vi "Main-side_features.vi"() -> ()   [LabVIEW 2015]
uses:
  <vilib>/Analysis/baseanly.llb/Mean (DBL).vi
  <vilib>/Utility/file.llb/Read Delimited Spreadsheet (string).vi
  <vilib>/Utility/file.llb/Write Delimited Spreadsheet (string).vi
  <vilib>/vision/NI_Vision_Development_Module.lvlib
  PlantType.dll
  TotalContoursConvexHull.dll
  2-top_features_oilseed/HistProperty.dll
  <vilib>/Analysis/NI_AALBase.lvlib
panel:
  in  "title-Path":path=path "H:/3-side_features_oilseed/title.txt"
  out "Gray Image":T1(plugin-control)
  out "savePath":path
  out "appended array":string[](array[string])
  out "im_width":i32
  out "im_height":i32
  in  "Date Path":path=path "H:/3-side_features_oilseed/rape_test/path.txt"
  out "Current Path":path
  out "Current Number":string
  out "Rotated Image":T1(plugin-control)
  out "HistStat_whole":dbl[](array[numeric])
  out "PAR (perimeter-to-area ratio)":dbl
  out "SFD":sgl
  out "BW (minimum circumscribed box width)":dbl
  out "BH (minimum circumscribed box height)":dbl
  out "TPA (Total projective area)":dbl
  out "R (Rectangularity)":dbl
  out "IFD":sgl
  out "Hull area":dbl
  out "AC (Area Convexity)":dbl
  out "HWR":dbl
  in  "ROI_flower":T2={"Top"=0, "im_height"=1450, "L_left"=0, "im_width"=1680}
  out "NB (Number of blanchs)":i32
  out "FPAR (Flower perimeter-to-area ratio)":dbl
  out "FSFD":sgl
  out "FBW (Flower minimum circumscribed box width)":dbl
  out "FBH (Flower minimum circumscribed box height)":dbl
  out "YPA (Yellow projective area)":dbl
  out "FR (Flower rectangularity)":dbl
  out "FIFD":sgl
  out "FAC (Flower area Convexity)":dbl
  out "HistStat_flower":dbl[](array[numeric])
  in  "ROI_whole":T2={"Top"=90, "im_height"=1970, "L_left"=300, "im_width"=1450}
  out "FHWR":dbl
  out "GPA (Green projective area)":dbl
  out "GPAR (Green / Total)":dbl
  out "YPAR (Yellow / Total)":dbl
  out "Flower Hull Image":T1(plugin-control)
  out "Flower Hull Area":dbl
  out "Cropped Image":T1(plugin-control)
  out "Binary Image":T1(plugin-control)
  out "rgb Hull Image":T1(plugin-control)
  out "Flower Image (RGB)":T1(plugin-control)
  out "Flower Image (Label)":T1(plugin-control)
  out "PD1-6":sgl[](array[numeric])
  out "f array":dbl[](array[numeric])
  out "Combined Image":T1(plugin-control)
  out "Image Path":path
  in  "Image Main Path":path=path "H:/3-side_features_oilseed/rape_test"
  # "Digital evaluation software for oilseed rape \nphenotype-related traits (side-view)"
  # "测量数据"
  # "Whole plant"
  # "均值"
  # "标准差"
  # "平滑度"
  # "三阶矩"
  # "一致性"
  # "熵"
  # "Flower"
  # "Ratio"
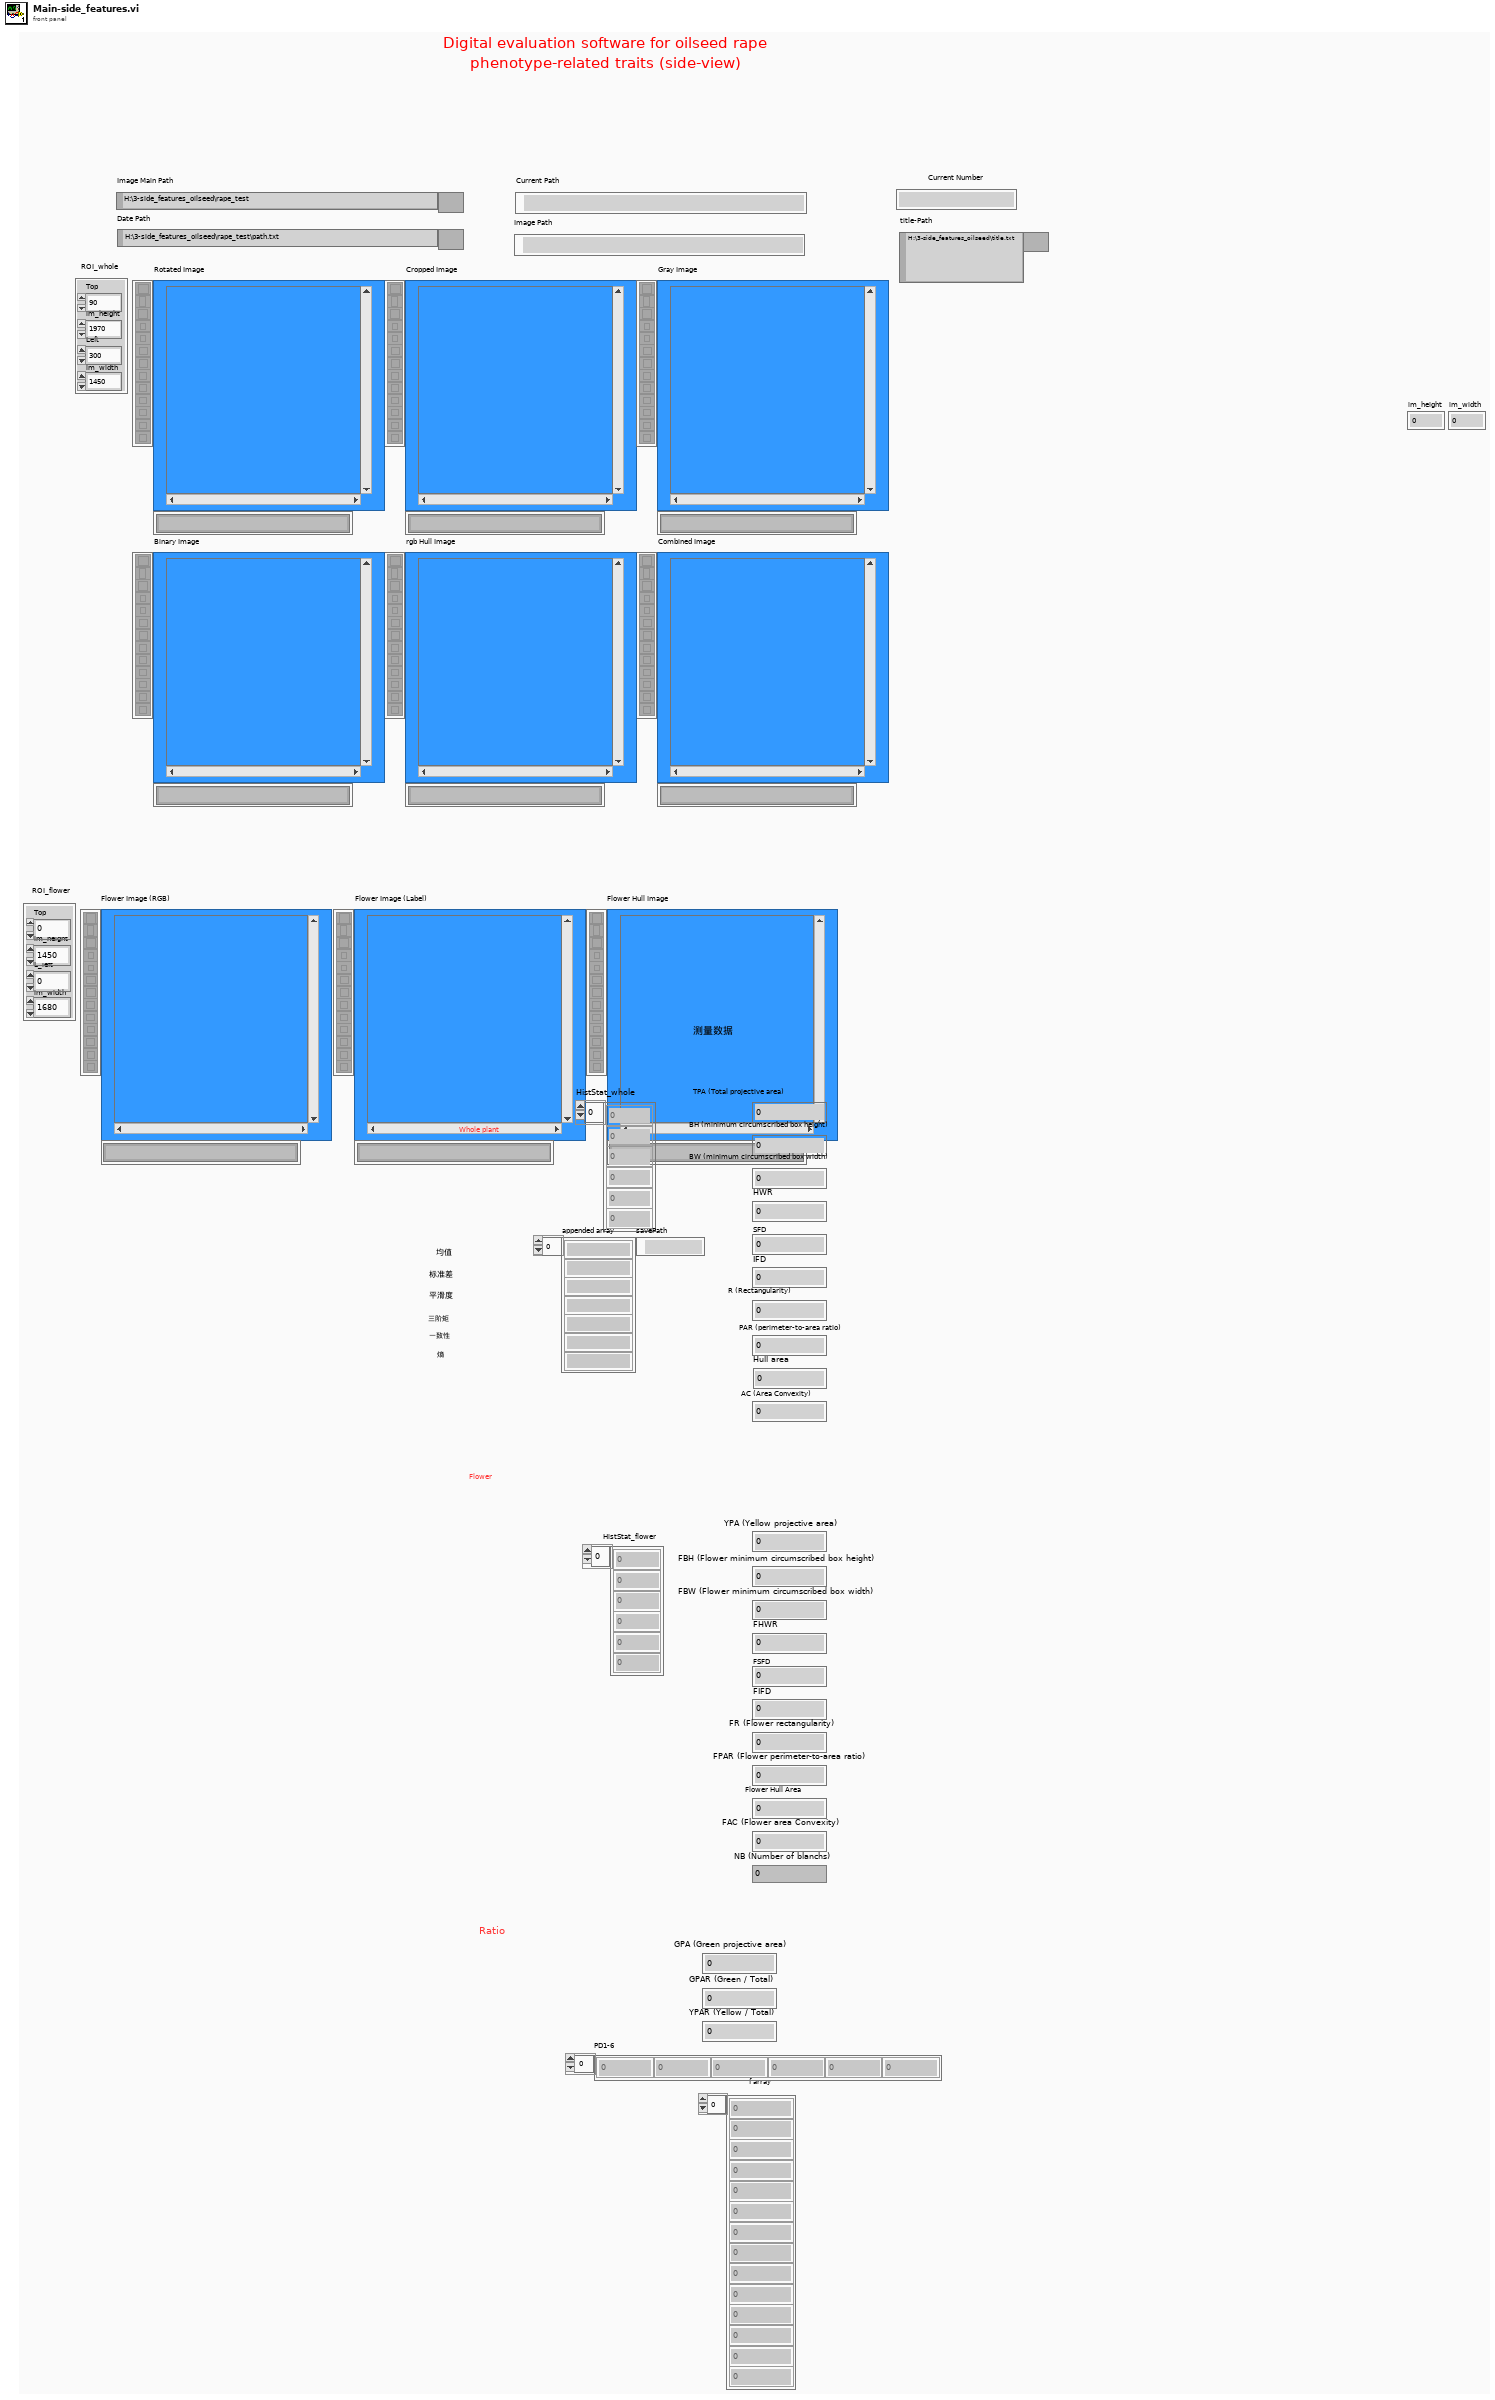
[diagram p1: front panel]
types:
  T1 = typedef "IMAQ Image.ctl" = refnum<image>
  T2 = cluster{"Top":i32, "im_height":i32, "L_left":i32, "im_width":i32}
  T3 = typedef "Image Type" = u32
  T4 = typedef "Particle Parameters" = i32
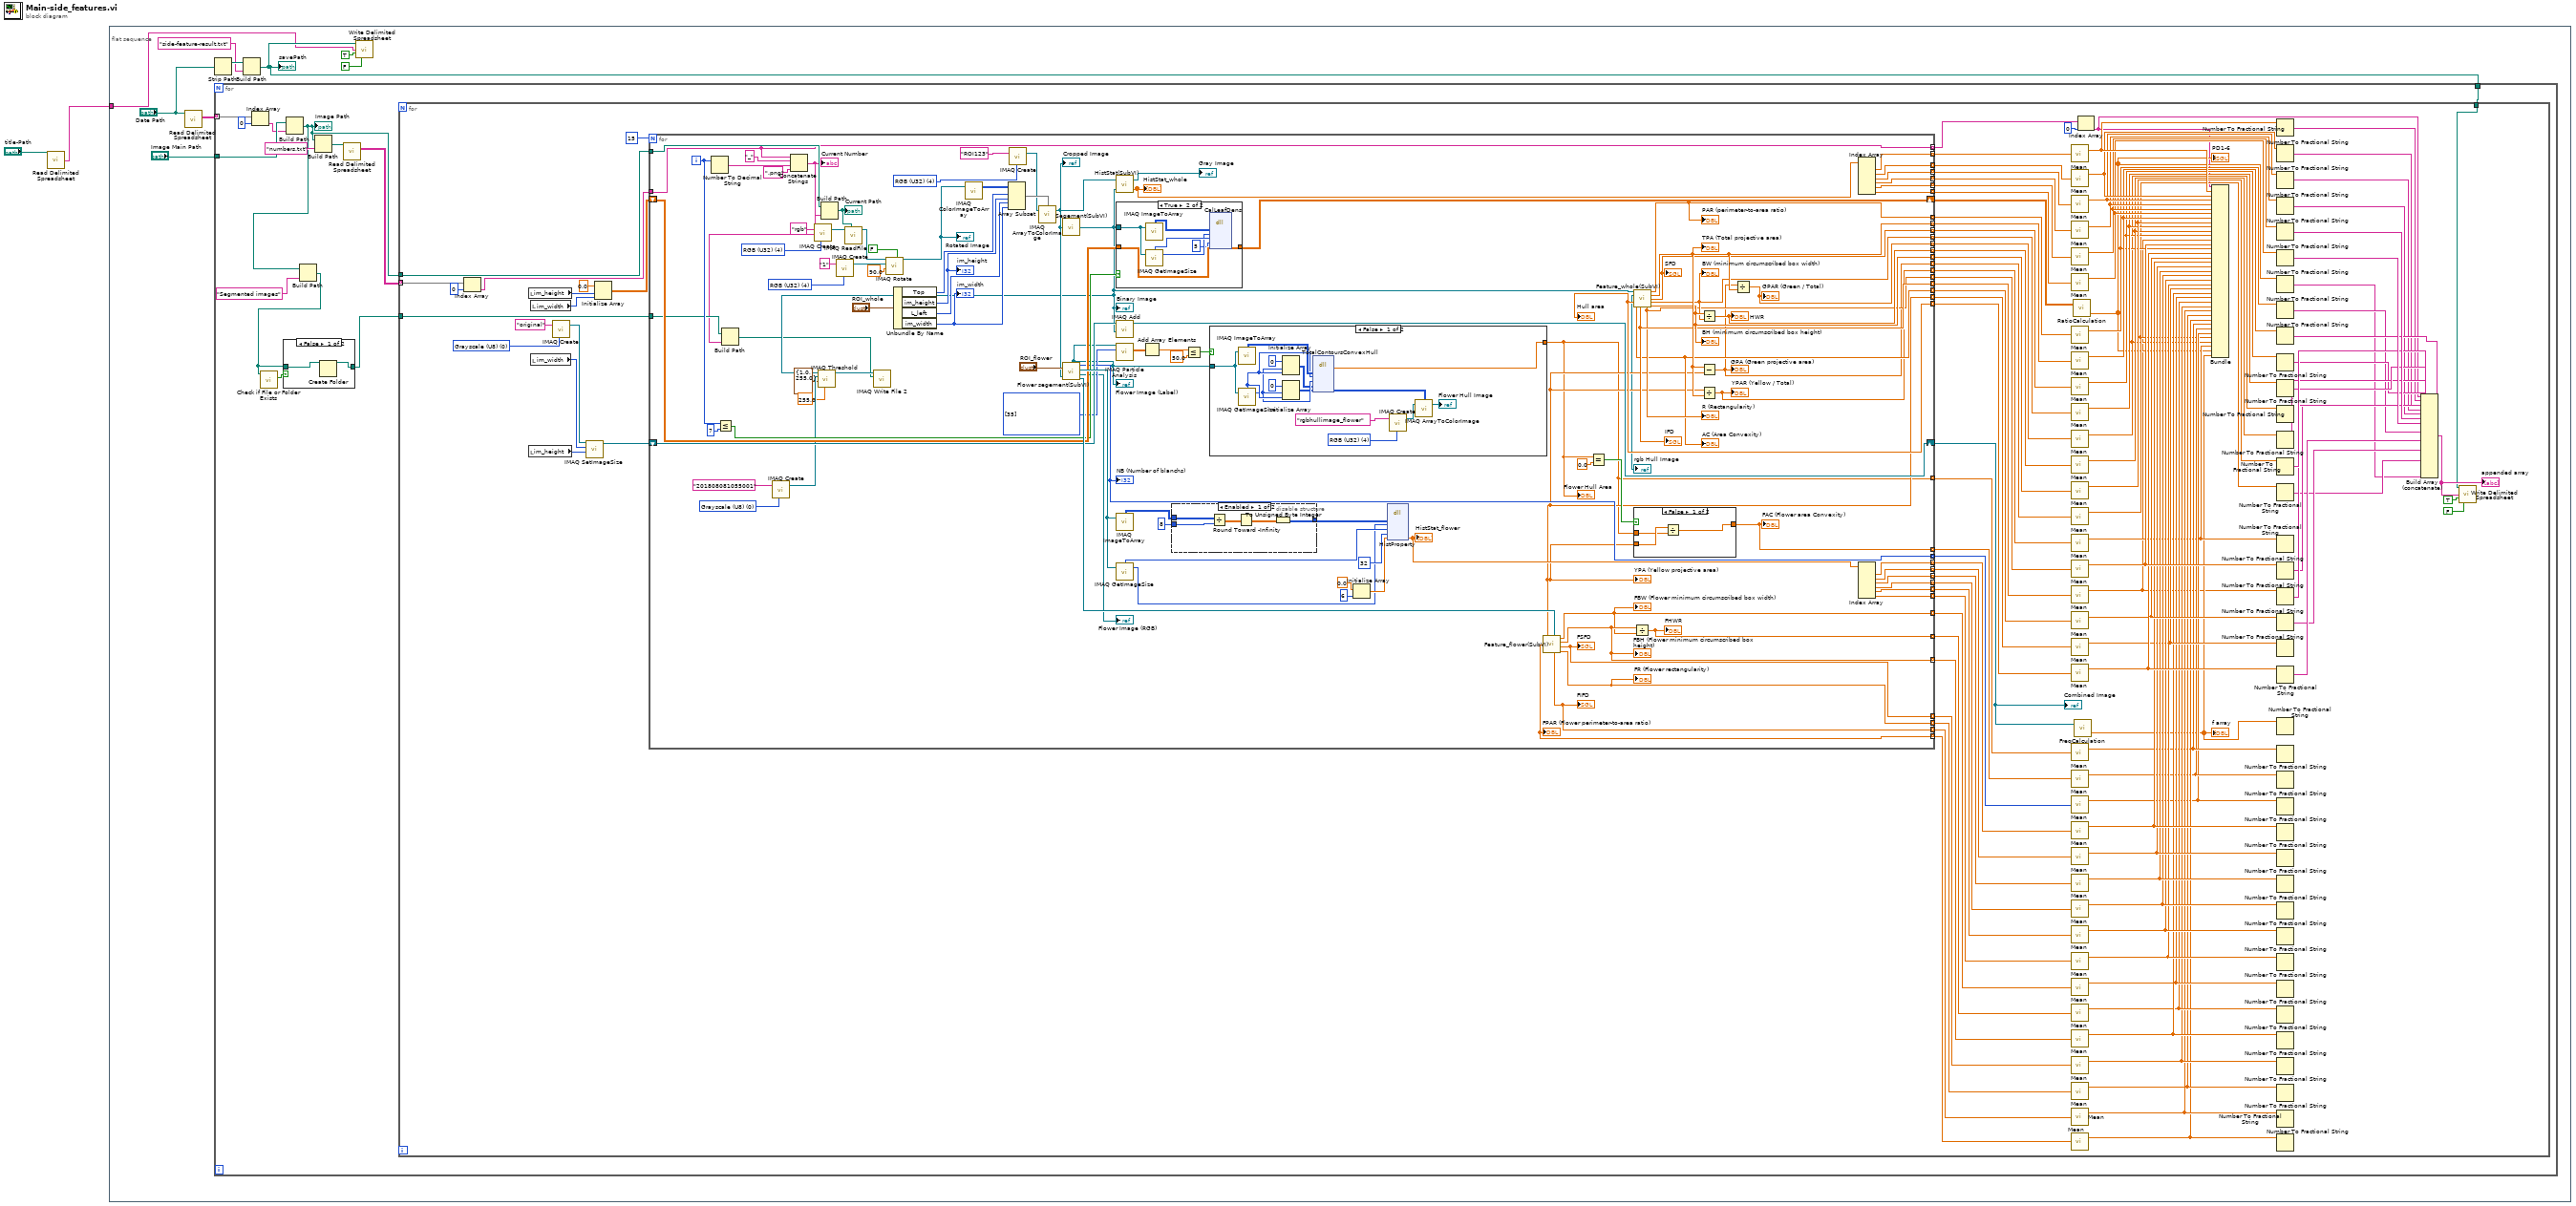
[diagram p0: block diagram]
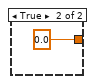
[diagram p3: hidden frame]
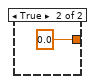
[diagram p4: hidden frame]
diagram:
  n1 = call-poly <vilib>:"Read Delimited Spreadsheet.vi"("file path (dialog if empty)"="title-Path") -> ("first row"=w1:string[])  [unwired: 9 in, 5 out]
  n2 = flat-sequence {
    tunnel: w1 -> [w3]
    frame #0 {
      n3 = call-poly <vilib>:"Read Delimited Spreadsheet.vi"("file path (dialog if empty)"="Date Path") -> ("all rows"=w10:string[][])  [unwired: 9 in, 5 out]
      n4 = Strip Path(path="Date Path") -> (stripped path=w8:path)  [unwired: 1 out]
      n5 = Build Path(base path=w8, name or relative path="side-feature-result.txt") -> (appended path=w4:path)
      "savePath" <- w4
      n6 = for {
        tunnel: "Image Main Path" -> [w24]
        tunnel: w10 -> [w22] mode=indexing
        tunnel: w4 -> [w17]
        n7 = Index Array(array=w22, index=0) -> (element=w19:string)
        n8 = Build Path(base path=w24, name or relative path=w19) -> (appended path=w16:path)
        "Image Path" <- w16
        n9 = Build Path(base path=w16, name or relative path="Segmented images") -> (appended path=w13:path)
        n10 = call <vilib>:"Check if File or Folder Exists.vi"("path"=w13) -> ("file or folder exists?"=w14:bool)  [unwired: 8 in, 2 out]
        n11 = case shown="False" w14 {
          tunnel: [w25 w27] -> w12
          tunnel: w13 -> [w26 w27]
          frame False {
            n12 = Create Folder(path (use dialog)=w26) -> (created path=w25:path)  [unwired: 2 in, 2 out]
          }
          frame True {
          }
        }
        n13 = Build Path(base path=w16, name or relative path="numbers.txt") -> (appended path=w20:path)
        n14 = call-poly <vilib>:"Read Delimited Spreadsheet.vi"("file path (dialog if empty)"=w20) -> ("all rows"=w18:string[][])  [unwired: 9 in, 5 out]
        n15 = for {
          tunnel: w16 -> [w142]
          tunnel: w18 -> [w143] mode=indexing
          tunnel: w17 -> [w32]
          tunnel: w12 -> [w31]
          w134 = T3 0 items=["Grayscale (U8)", "Grayscale (I16)", "Grayscale (SGL)", "Complex (CSG)", "RGB (U32)", "HSL (U32)", "RGB (U64)", "Grayscale (U16)"] ("Image Type")
          n16 = Index Array(array=w143, index=0) -> (element=w141:string)
          n17 = local read "im_height"() -> (w93:i32)
          n18 = local read "im_height"() -> (w92:i32)
          n19 = local read "im_width"() -> (w91:i32)
          n20 = local read "im_width"() -> (w90:i32)
          n21 = call "IMAQ Create"("Image Name"="original", "Image Type"=w134) -> ("New Image"=w135:T1)  [unwired: 2 in, 2 out]
          n22 = call "IMAQ SetImageSize"("Y Resolution"=w92, "X Resolution"=w90, "Image"=w135) -> ("Image Out"=w133:T1)  [unwired: 1 in, 2 out]
          n23 = Initialize Array(sgl 0.0 ("element"), w93, w91) -> (w138:sgl[][])
          n24 = for {
            N: 15 -> [_]
            tunnel: w142 -> [w242]
            tunnel: w141 -> [w157]
            shift-right: [w209] -> w137
            shift-left: w138 -> [w212]
            shift-right: [w207] -> w96
            shift-left: w133 -> [w208]
            tunnel: [w205] -> w132 mode=indexing
            tunnel: [w204] -> w131 mode=indexing
            tunnel: [w203] -> w130 mode=indexing
            tunnel: [w202] -> w129 mode=indexing
            tunnel: [w201] -> w128 mode=indexing
            tunnel: [w200] -> w127 mode=indexing
            tunnel: [w199] -> w126 mode=indexing
            tunnel: [w198] -> w125 mode=indexing
            tunnel: [w197] -> w124 mode=indexing
            tunnel: [w196] -> w123 mode=indexing
            tunnel: [w195] -> w122 mode=indexing
            tunnel: [w194] -> w121 mode=indexing
            tunnel: [w193] -> w120 mode=indexing
            tunnel: [w192] -> w119 mode=indexing
            tunnel: [w191] -> w118 mode=indexing
            tunnel: [w190] -> w117 mode=indexing
            tunnel: [w188] -> w116 mode=indexing
            tunnel: [w187] -> w115 mode=indexing
            tunnel: [w186] -> w114 mode=indexing
            tunnel: [w185] -> w113 mode=indexing
            tunnel: [w184] -> w112 mode=indexing
            tunnel: [w183] -> w111 mode=indexing
            tunnel: [w164] -> w110 mode=indexing
            tunnel: [w182] -> w109 mode=indexing
            tunnel: [w181] -> w108 mode=indexing
            tunnel: [w180] -> w107 mode=indexing
            tunnel: [w179] -> w106 mode=indexing
            tunnel: [w178] -> w105 mode=indexing
            tunnel: [w177] -> w104 mode=indexing
            tunnel: [w176] -> w103 mode=indexing
            tunnel: [w163] -> w102 mode=indexing
            tunnel: [w162] -> w101 mode=indexing
            tunnel: [w175] -> w100 mode=indexing
            tunnel: [w174] -> w99 mode=indexing
            tunnel: [w173] -> w98 mode=indexing
            tunnel: [w172] -> w97 mode=indexing
            tunnel: [w157] -> w95 mode=indexing
            tunnel: w31 -> [w154]
            i -> [w156]
            w150 = u32 0 items=["Grayscale (U8)", "Grayscale (I16)", "Grayscale (SGL)", "Complex (CSG)", "RGB (U32)", "HSL (U32)", "RGB (U64)"] ("Image Type")
            w171 = T4[] [35] items=["Center of Mass X", "Center of Mass Y", "First Pixel X", "First Pixel Y", "Bounding Rect Left", "Bounding Rect Top", "Bounding Rect Right", "Bounding Rect Bottom", "Max Feret Diameter Start X", "Max Feret Diameter Start Y", "Max Feret Diameter End X", "Max Feret Diameter End Y", "Max Horiz. Segment Length Left", "Max Horiz. Segment Length Right", "Max Horiz. Segment Length Row", "-", "Bounding Rect Width", "Bounding Rect Height", "Bounding Rect Diagonal", "Perimeter", "Convex Hull Perimeter", "Holes' Perimeter", "Max Feret Diameter", "Equivalent Ellipse Major Axis", "Equivalent Ellipse Minor Axis", "Equivalent Ellipse Minor Axis (Feret)", "Equivalent Rect Long Side", "Equivalent Rect Short Side", "Equivalent Rect Diagonal", "Equivalent Rect Short Side (Feret)", "Average Horiz. Segment Length", "Average Vert. Segment Length", "Hydraulic Radius", "Waddel Disk Diameter", "-", "Area", "Holes' Area", "Particle & Holes' Area", "Convex Hull Area", "Image Area", "-", "Number of Holes", "Number of Horiz. Segments", "Number of Vert. Segments", "-", "Orientation", "Max Feret Diameter Orientation", "-", "% Area/Image Area", "% Area/(Particle & Holes' Area)", "Ratio of Equivalent Ellipse Axes", "Ratio of Equivalent Rect Sides", "-", "Elongation Factor", "Compactness Factor", "Heywood Circularity Factor", "Type Factor", "-", "Sum X", "Sum Y", "Sum XX", "Sum XY", "Sum YY", "Sum XXX", "Sum XXY", "Sum XYY", "Sum YYY", "-", "Moment of Inertia XX", "Moment of Inertia XY", "Moment of Inertia YY", "Moment of Inertia XXX", "Moment of Inertia XXY", "Moment of Inertia XYY", "Moment of Inertia YYY", "Norm. Moment of Inertia XX", "Norm. Moment of Inertia XY", "Norm. Moment of Inertia YY", "Norm. Moment of Inertia XXX", "Norm. Moment of Inertia XXY", "Norm. Moment of Inertia XYY", "Norm. Moment of Inertia YYY", "Hu Moment 1", "Hu Moment 2", "Hu Moment 3", "Hu Moment 4", "Hu Moment 5", "Hu Moment 6", "Hu Moment 7"] ("Pixel Measurements")
            w228 = u32 4 items=["Grayscale (U8)", "Grayscale (I16)", "Grayscale (SGL)", "Complex (CSG)", "RGB (U32)", "HSL (U32)", "RGB (U64)"] ("Image Type")
            w240 = T3 4 items=["Grayscale (U8)", "Grayscale (I16)", "Grayscale (SGL)", "Complex (CSG)", "RGB (U32)", "HSL (U32)", "RGB (U64)", "Grayscale (U16)"] ("Image Type")
            w247 = T3 4 items=["Grayscale (U8)", "Grayscale (I16)", "Grayscale (SGL)", "Complex (CSG)", "RGB (U32)", "HSL (U32)", "RGB (U64)", "Grayscale (U16)"] ("Image Type")
            n25 = Number To Decimal String(number=w156) -> (decimal integer string=w244:string)  [unwired: 1 out]
            n26 = Less Or Equal?(x=w156, y=u32 7) -> (x <= y?=w210:bool)
            n27 = call "IMAQ Create"("Image Name"="201808081055001", "Image Type"=w150) -> ("New Image"=w149:T1)  [unwired: 2 in, 2 out]
            n28 = Concatenate Strings(w157, "_" ("string"), w244, ".png" ("string")) -> (w153:string)
            "Current Number" <- w153
            n29 = Build Path(base path=w154, name or relative path=w153) -> (appended path=w145:path)
            n30 = call "IMAQ Create"("Image Name"="rgb", "Image Type"=w247) -> ("New Image"=w248:T1)  [unwired: 2 in, 2 out]
            n31 = Build Path(base path=w242, name or relative path=w153) -> (appended path=w243:path)
            "Current Path" <- w243
            n32 = call "IMAQ Create"("Image Name"="1", "Image Type"=w240) -> ("New Image"=w238:T1)  [unwired: 2 in, 2 out]
            n33 = call "IMAQ ReadFile"("File Path"=w243, "Image"=w248) -> ("Image Out"=w236:T1)  [unwired: 3 in, 6 out]
            n34 = call "IMAQ Rotate"("Maintain Size"=FALSE, "Angle (degrees)"=sgl 90.0, "Image Dst"=w238, "Image Src"=w236) -> ("Image Dst Out"=w226:T1)  [unwired: 4 in, 3 out]
            "Rotated Image" <- w226
            n35 = Unbundle By Name("ROI_whole") -> ("Top"=w232:i32, "im_height"=w233:i32, "L_left"=w234:i32, "im_width"=w235:i32)
            "im_height" <- w233
            "im_width" <- w235
            n36 = call "IMAQ ColorImageToArray"("Image"=w226) -> ("Image Pixels (U32)"=w231:u32[][])  [unwired: 2 in, 3 out]
            n37 = Array Subset(array=w231, index (row)=w232, length (row)=w233, index (col)=w234, length (col)=w235) -> (w230:u32[][])
            n38 = call "IMAQ Create"("Image Name"="ROI123", "Image Type"=w228) -> ("New Image"=w227:T1)  [unwired: 2 in, 2 out]
            n39 = call "IMAQ ArrayToColorImage"("Image Pixels (U32)"=w230, "Image"=w227) -> ("Image Out"=w161:T1)  [unwired: 2 in, 2 out]
            "Cropped Image" <- w161
            n40 = call "Segement(SubVI).vi"("Image in"=w161) -> ("Binary Image"=w152:T1)
            "Binary Image" <- w152
            n41 = call "IMAQ Threshold"("Replace Value"=sgl 255.0, "Range"=cluster{"Lower value":sgl, "Upper value":sgl} {"Lower value"=1.0, "Upper value"=255.0}, "Image Dst"=w149, "Image Src"=w152) -> ("Image Dst Out"=w146:T1)  [unwired: 6 in, 1 out]
            n42 = call-poly "IMAQ Write File 2"("File Path"=w145, "Image"=w146) -> ()  [unwired: 8 in, 2 out]
            n43 = call "Flower segement(SubVI).vi"("Image in"=w161, "ROI 上半部分 2"="ROI_flower") -> ("黄色分量（油菜花）二值图"=w224:T1, "黄色分量（油菜花）"=→"Flower Image (RGB)":T1, "黄色分量（油菜花）Gray"=w214:T1, "Number of Particles"=w175:i32, "RGB花标记"=w158:T1)
            "NB (Number of blanchs)" <- w175
            "Flower Image (Label)" <- w158
            n44 = call "HistStat(SubVI).vi"("Binary Image"=w152, "Original Image"=w161) -> ("HistStat"=w206:dbl[], "Gray Image"=→"Gray Image":T1)
            "HistStat_whole" <- w206
            n45 = case shown="True" w210 {
              tunnel: w152 -> [_ w273]
              tunnel: w212 -> [w269 w272]
              tunnel: [w269 w271] -> w209
              frame False {
              }
              frame True {
                n46 = call "IMAQ ImageToArray"("Image"=w273) -> ("Image Pixels (U8)"=w276:u8[][])  [unwired: 2 in, 5 out]
                n47 = call "IMAQ GetImageSize"("Image"=w273) -> ("Y Resolution"=w274:i32, "X Resolution"=w275:i32)  [unwired: 1 in, 3 out]
                n48 = dll-call lib="H:/3-side_features_oilseed/PlantType.dll" fn="CalLeafDens"("bw"=w276, "row"=w274, "col"=w275, "GridSize"=5, "dens"=w272) -> ("dens"=w271:sgl[][])  [unwired: 7 in, 3 out]
              }
            }
            n49 = call "IMAQ Add"("Image Src A"=w208, "Image Src B"=w152) -> ("Image Dst Out"=w207:T1)  [unwired: 3 in, 3 out]
            n50 = call "IMAQ Particle Analysis"("Pixel Measurements"=w171, "Image"=w158) -> ("Particle Measurements (Pixels)"=w170:dbl[][])  [unwired: 3 in, 6 out]
            n51 = call "IMAQ ImageToArray"("Image"=w214) -> ("Image Pixels (U8)"=w215:u8[][])  [unwired: 2 in, 5 out]
            n52 = call "IMAQ GetImageSize"("Image"=w214) -> ("Y Resolution"=w218:i32, "X Resolution"=w219:i32)  [unwired: 1 in, 3 out]
            n53 = Add Array Elements(numeric array=w170) -> (sum=w169:dbl)
            n54 = disable-structure shown="Enabled" {
              disable-tunnel: w215 -> [w281 w282]
              disable-tunnel: u8 8 ("y") -> [w280 _]
              disable-tunnel: [w277 w282] -> w217
              frame Enabled {
                n55 = Divide(x=w281, y=w280) -> (x/y=w279:dbl[][])
                n56 = Round Toward -Infinity(1:w279) -> (0:w278:dbl[][])
                n57 = To Unsigned Byte Integer(number=w278) -> (unsigned 8bit integer=w277:u8[][])
              }
              frame Disabled {
              }
            }
            n58 = Less Or Equal?(x=w169, y=50.0) -> (x <= y?=w167:bool)
            n59 = case shown="False" w167 {
              tunnel: w158 -> [w256 _]
              tunnel: [w255 0.0 ("areaSum")] -> w163
              frame False {
                w262 = T3 4 items=["Grayscale (U8)", "Grayscale (I16)", "Grayscale (SGL)", "Complex (CSG)", "RGB (U32)", "HSL (U32)", "RGB (U64)", "Grayscale (U16)"] ("Image Type")
                n60 = call "IMAQ ImageToArray"("Image"=w256) -> ("Image Pixels (U8)"=w267:u8[][])  [unwired: 2 in, 5 out]
                n61 = call "IMAQ GetImageSize"("Image"=w256) -> ("Y Resolution"=w265:i32, "X Resolution"=w266:i32)  [unwired: 1 in, 3 out]
                n62 = Initialize Array(u8 0 ("element"), w265, w266) -> (w257:u8[][])
                n63 = Initialize Array(u32 0 ("element"), w265, w266) -> (w260:u32[][])
                n64 = dll-call lib="H:/3-side_features_oilseed/TotalContoursConvexHull.dll" fn="TotalContoursConvexHull"("src"=w267, "width"=w266, "height"=w265, "bwhullimage"=w257, "rgbhullimage"=w260) -> ("areaSum"=w255:dbl, "rgbhullimage"=w263:u32[][])  [unwired: 7 in, 2 out]
                n65 = call "IMAQ Create"("Image Name"="rgbhullimage_flower", "Image Type"=w262) -> ("New Image"=w264:T1)  [unwired: 2 in, 2 out]
                n66 = call "IMAQ ArrayToColorImage"("Image Pixels (U32)"=w263, "Image"=w264) -> ("Image Out"=→"Flower Hull Image":T1)  [unwired: 2 in, 2 out]
              }
              frame True {
              }
            }
            "Flower Hull Area" <- w163
            n67 = Initialize Array(0.0 ("element"), 6 ("dimension size")) -> (w222:dbl[])
            n68 = dll-call lib="H:/2-top_features_oilseed/HistProperty.dll" fn="HistProperty"("Im"=w217, "row"=w218, "col"=w219, "G"=32, "HistStat"=w222) -> ("HistStat"=w189:dbl[])  [unwired: 7 in, 3 out]
            "HistStat_flower" <- w189
            n69 = call "Feature_flower(SubVI).vi"("黄色分量（油菜花）二值图"=w224) -> ("SF 3"=w177:dbl, "IFD 2"=w178:sgl, "SFD 2"=w179:sgl, "SH 2"=w182:dbl, "SW 2"=w181:dbl, "SE 2"=w176:dbl, "SA"=w164:dbl)  [unwired: 1 out]
            "FPAR (Flower perimeter-to-area ratio)" <- w176
            "FSFD" <- w179
            "FBW (Flower minimum circumscribed box width)" <- w181
            "FBH (Flower minimum circumscribed box height)" <- w182
            "YPA (Yellow projective area)" <- w164
            "FR (Flower rectangularity)" <- w177
            "FIFD" <- w178
            n70 = Equal?(x=w163, y=0.0) -> (x = y?=w166:bool)
            n71 = Divide(x=w182, y=w181) -> (x/y=w180:dbl)
            "FHWR" <- w180
            n72 = call "Feature_whole(SubVI).vi"("Binary Image"=w152) -> ("SE"=w192:dbl, "rgb Hull Image 2"=→"rgb Hull Image":T1, "SA"=w199:dbl, "SFD"=w195:sgl, "Hull area"=w191:dbl, "SW"=w197:dbl, "SF 2"=w190:dbl, "IFD"=w194:sgl, "SF"=w193:dbl, "SH"=w198:dbl)  [unwired: 5 out]
            "PAR (perimeter-to-area ratio)" <- w192
            "SFD" <- w195
            "BW (minimum circumscribed box width)" <- w197
            "BH (minimum circumscribed box height)" <- w198
            "TPA (Total projective area)" <- w199
            "R (Rectangularity)" <- w193
            "IFD" <- w194
            "Hull area" <- w191
            "AC (Area Convexity)" <- w190
            n73 = case shown="False" w166 {
              tunnel: w164 -> [w252 _]
              tunnel: w163 -> [w251 _]
              tunnel: [w250 0.0] -> w162
              frame False {
                n74 = Divide(x=w252, y=w251) -> (x/y=w250:dbl)
              }
              frame True {
              }
            }
            "FAC (Flower area Convexity)" <- w162
            n75 = Divide(x=w198, y=w197) -> (x/y=w196:dbl)
            "HWR" <- w196
            n76 = Subtract(x=w199, y=w164) -> (x-y=w174:dbl)
            "GPA (Green projective area)" <- w174
            n77 = Divide(x=w164, y=w199) -> (x/y=w172:dbl)
            "YPAR (Yellow / Total)" <- w172
            n78 = Divide(x=w174, y=w199) -> (x/y=w173:dbl)
            "GPAR (Green / Total)" <- w173
            n79 = Index Array(array=w206) -> (element #1=w205:dbl, element #2=w204:dbl, element #3=w203:dbl, element #4=w202:dbl, element #5=w201:dbl, element #6=w200:dbl)  [unwired: 6 in]
            n80 = Index Array(array=w189) -> (element #1=w188:dbl, element #2=w187:dbl, element #3=w186:dbl, element #4=w185:dbl, element #5=w184:dbl, element #6=w183:dbl)  [unwired: 6 in]
          }
          "Combined Image" <- w96
          n81 = call-poly <vilib>:"Mean.vi"("X"=w132) -> ("mean"=w89:dbl)  [unwired: 1 out]
          n82 = call-poly <vilib>:"Mean.vi"("X"=w131) -> ("mean"=w88:dbl)  [unwired: 1 out]
          n83 = call-poly <vilib>:"Mean.vi"("X"=w130) -> ("mean"=w87:dbl)  [unwired: 1 out]
          n84 = call-poly <vilib>:"Mean.vi"("X"=w129) -> ("mean"=w86:dbl)  [unwired: 1 out]
          n85 = call-poly <vilib>:"Mean.vi"("X"=w128) -> ("mean"=w85:dbl)  [unwired: 1 out]
          n86 = call-poly <vilib>:"Mean.vi"("X"=w127) -> ("mean"=w84:dbl)  [unwired: 1 out]
          n87 = call-poly <vilib>:"Mean.vi"("X"=w119) -> ("mean"=w77:dbl)  [unwired: 1 out]
          n88 = call-poly <vilib>:"Mean.vi"("X"=w126) -> ("mean"=w83:dbl)  [unwired: 1 out]
          n89 = call-poly <vilib>:"Mean.vi"("X"=w122) -> ("mean"=w79:dbl)  [unwired: 1 out]
          n90 = call-poly <vilib>:"Mean.vi"("X"=w124) -> ("mean"=w81:dbl)  [unwired: 1 out]
          n91 = call-poly <vilib>:"Mean.vi"("X"=w98) -> ("mean"=w56:dbl)  [unwired: 1 out]
          n92 = call-poly <vilib>:"Mean.vi"("X"=w123) -> ("mean"=w80:dbl)  [unwired: 1 out]
          n93 = call-poly <vilib>:"Mean.vi"("X"=w125) -> ("mean"=w82:dbl)  [unwired: 1 out]
          n94 = call-poly <vilib>:"Mean.vi"("X"=w99) -> ("mean"=w57:dbl)  [unwired: 1 out]
          n95 = call-poly <vilib>:"Mean.vi"("X"=w97) -> ("mean"=w55:dbl)  [unwired: 1 out]
          n96 = call-poly <vilib>:"Mean.vi"("X"=w120) -> ("mean"=w78:dbl)  [unwired: 1 out]
          n97 = call-poly <vilib>:"Mean.vi"("X"=w121) -> ("mean"=w28:dbl)  [unwired: 1 out]
          n98 = call-poly <vilib>:"Mean.vi"("X"=w117) -> ("mean"=w75:dbl)  [unwired: 1 out]
          n99 = call-poly <vilib>:"Mean.vi"("X"=w110) -> ("mean"=w68:dbl)  [unwired: 1 out]
          n100 = call-poly <vilib>:"Mean.vi"("X"=w118) -> ("mean"=w76:dbl)  [unwired: 1 out]
          n101 = call-poly <vilib>:"Mean.vi"("X"=w102) -> ("mean"=w60:dbl)  [unwired: 1 out]
          n102 = call-poly <vilib>:"Mean.vi"("X"=w101) -> ("mean"=w59:dbl)  [unwired: 1 out]
          n103 = call-poly <vilib>:"Mean.vi"("X"=w100) -> ("mean"=w58:dbl)  [unwired: 1 out]
          n104 = call-poly <vilib>:"Mean.vi"("X"=w116) -> ("mean"=w74:dbl)  [unwired: 1 out]
          n105 = call-poly <vilib>:"Mean.vi"("X"=w115) -> ("mean"=w73:dbl)  [unwired: 1 out]
          n106 = call-poly <vilib>:"Mean.vi"("X"=w114) -> ("mean"=w72:dbl)  [unwired: 1 out]
          n107 = call-poly <vilib>:"Mean.vi"("X"=w113) -> ("mean"=w71:dbl)  [unwired: 1 out]
          n108 = call-poly <vilib>:"Mean.vi"("X"=w112) -> ("mean"=w70:dbl)  [unwired: 1 out]
          n109 = call-poly <vilib>:"Mean.vi"("X"=w111) -> ("mean"=w69:dbl)  [unwired: 1 out]
          n110 = call-poly <vilib>:"Mean.vi"("X"=w108) -> ("mean"=w66:dbl)  [unwired: 1 out]
          n111 = call-poly <vilib>:"Mean.vi"("X"=w107) -> ("mean"=w65:dbl)  [unwired: 1 out]
          n112 = call-poly <vilib>:"Mean.vi"("X"=w109) -> ("mean"=w67:dbl)  [unwired: 1 out]
          n113 = call-poly <vilib>:"Mean.vi"("X"=w106) -> ("mean"=w64:dbl)  [unwired: 1 out]
          n114 = call-poly <vilib>:"Mean.vi"("X"=w104) -> ("mean"=w62:dbl)  [unwired: 1 out]
          n115 = call-poly <vilib>:"Mean.vi"("X"=w105) -> ("mean"=w63:dbl)  [unwired: 1 out]
          n116 = call-poly <vilib>:"Mean.vi"("X"=w103) -> ("mean"=w61:dbl)  [unwired: 1 out]
          n117 = call "RatioCalculation.vi"("dens"=w137) -> ("ratio"=w54:sgl[])  [unwired: 2 out]
          "PD1-6" <- w54
          n118 = call "FreqCalculation.vi"("Acc Image"=w96) -> ("f array"=w53:dbl[])  [unwired: 2 out]
          "f array" <- w53
          n119 = Index Array(array=w95, index=0) -> (element=w40:string)
          n120 = Bundle("String"=w40, "mean"=w89, "mean"=w88, "mean"=w87, "mean"=w86, "mean"=w85, "mean"=w84, "mean"=w83, "mean"=w82, "mean"=w81, "mean"=w80, "mean"=w79, "mean"=w28, "mean"=w78, "mean"=w77, "mean"=w76, "mean"=w75, "mean"=w74, "mean"=w73, "mean"=w72, "mean"=w71, "mean"=w70, "mean"=w69, "mean"=w68, "mean"=w67, "mean"=w66, "mean"=w65, "mean"=w64, "mean"=w63, "mean"=w62, "mean"=w61, "mean"=w60, "mean"=w59, "mean"=w58, "mean"=w57, "mean"=w56, "mean"=w55, "ratio"=w54, "f array"=w53) -> ()  [unwired: 1 in, 1 out]
          n121 = Number To Fractional String(number=w89) -> (F-format string=w39:string)  [unwired: 3 in]
          n122 = Number To Fractional String(number=w88) -> (F-format string=w38:string)  [unwired: 3 in]
          n123 = Number To Fractional String(number=w87) -> (F-format string=w37:string)  [unwired: 3 in]
          n124 = Number To Fractional String(number=w86) -> (F-format string=w36:string)  [unwired: 3 in]
          n125 = Number To Fractional String(number=w85) -> (F-format string=w52:string)  [unwired: 3 in]
          n126 = Number To Fractional String(number=w84) -> (F-format string=w51:string)  [unwired: 3 in]
          n127 = Number To Fractional String(number=w54) -> (F-format string=w29:string[])  [unwired: 3 in]
          n128 = Number To Fractional String(number=w77) -> (F-format string=w43:string)  [unwired: 3 in]
          n129 = Number To Fractional String(number=w83) -> (F-format string=w50:string)  [unwired: 3 in]
          n130 = Number To Fractional String(number=w79) -> (F-format string=w46:string)  [unwired: 3 in]
          n131 = Number To Fractional String(number=w81) -> (F-format string=w48:string)  [unwired: 3 in]
          n132 = Number To Fractional String(number=w56) -> ()  [unwired: 3 in, 1 out]
          n133 = Number To Fractional String(number=w80) -> (F-format string=w47:string)  [unwired: 3 in]
          n134 = Number To Fractional String(number=w82) -> (F-format string=w49:string)  [unwired: 3 in]
          n135 = Number To Fractional String(number=w57) -> (F-format string=w30:string)  [unwired: 3 in]
          n136 = Number To Fractional String(number=w55) -> ()  [unwired: 3 in, 1 out]
          n137 = Number To Fractional String(number=w78) -> (F-format string=w44:string)  [unwired: 3 in]
          n138 = Number To Fractional String(number=w28) -> (F-format string=w45:string)  [unwired: 3 in]
          n139 = Number To Fractional String(number=w75) -> (F-format string=w41:string)  [unwired: 3 in]
          n140 = Number To Fractional String(number=w68) -> ()  [unwired: 3 in, 1 out]
          n141 = Number To Fractional String(number=w76) -> (F-format string=w42:string)  [unwired: 3 in]
          n142 = Number To Fractional String(number=w53) -> ()  [unwired: 3 in, 1 out]
          n143 = Number To Fractional String(number=w60) -> ()  [unwired: 3 in, 1 out]
          n144 = Number To Fractional String(number=w59) -> ()  [unwired: 3 in, 1 out]
          n145 = Number To Fractional String(number=w58) -> ()  [unwired: 3 in, 1 out]
          n146 = Number To Fractional String(number=w74) -> ()  [unwired: 3 in, 1 out]
          n147 = Number To Fractional String(number=w73) -> ()  [unwired: 3 in, 1 out]
          n148 = Number To Fractional String(number=w72) -> ()  [unwired: 3 in, 1 out]
          n149 = Number To Fractional String(number=w71) -> ()  [unwired: 3 in, 1 out]
          n150 = Number To Fractional String(number=w70) -> ()  [unwired: 3 in, 1 out]
          n151 = Number To Fractional String(number=w69) -> ()  [unwired: 3 in, 1 out]
          n152 = Number To Fractional String(number=w66) -> ()  [unwired: 3 in, 1 out]
          n153 = Number To Fractional String(number=w65) -> ()  [unwired: 3 in, 1 out]
          n154 = Number To Fractional String(number=w67) -> ()  [unwired: 3 in, 1 out]
          n155 = Number To Fractional String(number=w64) -> ()  [unwired: 3 in, 1 out]
          n156 = Number To Fractional String(number=w62) -> ()  [unwired: 3 in, 1 out]
          n157 = Number To Fractional String(number=w63) -> ()  [unwired: 3 in, 1 out]
          n158 = Number To Fractional String(number=w61) -> ()  [unwired: 3 in, 1 out]
          n159 = Build Array (concatenate)(w40, w39, w38, w37, w36, w52, w51, w50, w49, w48, w47, w46, w45, w44, w43, w42, w41, w30, w29) -> (w35:string[])
          "appended array" <- w35
          n160 = call-poly <vilib>:"Write Delimited Spreadsheet.vi"("file path (dialog if empty)"=w32, "1D data"=w35, "append to file? (F)"=TRUE, "transpose? (F)"=FALSE) -> ()  [unwired: 10 in, 2 out]
        }
      }
      n161 = call-poly <vilib>:"Write Delimited Spreadsheet.vi"("file path (dialog if empty)"=w4, "1D data"=w3, "append to file? (F)"=TRUE, "transpose? (F)"=FALSE) -> ()  [unwired: 10 in, 2 out]
    }
  }
